vi "FTMS.vi"() -> ()   [LabVIEW 2012]
uses:
  Hardware Control/OSC/SubVIs/controls/sampling_rate.ctl
  Hardware Control/OSC/SubVIs/controls/scale.ctl
  global.vi
  <vilib>/Platform/browser.llb/Open URL in Default Browser (string).vi
panel:
  out "Meas Cycle \nDuration (s)":dbl=2.0 format="%.2g"
  out "Experiment \ncomplete in":string="00:00:00"
  out "Duration \nper Step":string="00:00:00"
  out "Time left for\ncurrent Step":string
  in  "about":bool
  in  "readme":bool
  out "Current Average":i32=2
  out "TRIG burst enable":bool=TRUE caption="Burst"
  out "TRIG inhibit off":dbl=0.000745 min=0.0 max=999.999999999995 format="%.1p"
  out "Writing File":bool
  out "OSC Reading":bool
  out "Waiting":bool
  out "Current Step":i32=4
  out "Current Center \nFrequency (Hz)":dbl=9000000000.0 format="%0.2p"
  in  "meas cluster":T1
  in  "Pause":bool
  in  "Stop":bool
  out "dt":dbl=2e-10 format="%#_6p"
  out "reset meas cycle timer":bool
  out "first start":bool
  in  "Tab Control":T2(tab)
  in  "Single Trigger":bool
  in  "EXP File Path":path=path "U:/Measurement Data" caption="Enter or select file path"
  in  "Safe Single Step Spectra":bool
  in  "Safe Single Step Time Signals":bool
  in  "Safe Combined Spectra":bool=TRUE
  in  "EXP Meas Period (s)":dbl=1.0 caption="Meas Period (s)" min=1.0 format="%.2g"
  in  "EXP Meas Cycles":i32=2 caption="Number of Averages" min=1 step=1
  out "Step Duration":string
  in  "Purge Freq.":dbl=2.0 caption="Purge Freq. (Hz)"
  in  "PURGE nozzle":bool
  out "TRIG BG cycle":dbl=0.001 caption="BG. cycle" min=0.0 max=999.999999999995 format="%.2p"
  out "TRIG mol delay":dbl=0.0006 caption="Mol. delay (s)" min=0.0 max=999.999999999995 format="%.2p"
  out "TRIG start time":dbl[](array[numeric])=[0.0, 1.1e-06, 6.6e-06, 6.4e-06] caption="Delay \nStarts (s)" format="%.3p"
  out "TRIG delay duration":dbl=4.7e-05 caption="Delay Cycle (s)" format="%.2p"
  out "TRIG duration":dbl[](array[numeric])=[5.65e-06, 5e-06, 4e-05, 5e-06] caption="Delay \nDurations (s)" min=0.0 format="%.3p"
  out "TRIG burst period":dbl=5e-05 caption="Burst Period (s)" format="%.2p"
  out "TRIG burst count":i32=3 caption="Bursts"
  in  "Refresh meas time":bool
  out "meas cycle time (ms)":u32
  out "OSC resolution":ext=25000.0 caption="Spectral Resolution (Hz)" format="%#_6p"
  out "OSC sample points":i32=200000 caption="Points / Frame"
  out "Horizontal Scale":T3=4e-06 items=["400ns/div"=4e-07, "1µs/div"=1e-06, "2µs/div"=2e-06, "4µs/div"=4e-06, "10µs/div"=1e-05, "20µs/div"=2e-05]
  out "meas duration (s)":dbl=3.9999999999999996e-05 format="%.1p"
  out "Sample Rate (Hz)":T4=5000000000.0 items=["20 GHz (50ps/sample)", "10 GHz (100ps/sample)", "5.0 GHz (200ps/sample)", "2.5 GHz (400ps/sample)", "1.25 GHz (0.8ns/sample)", "0.5 GHz (2ns/sample)"]
  in  "start experiment":bool
  in  "config TRIG":bool
  in  "config OSC":bool
  in  "PSG start freq":dbl=6000000000.0 caption="Start Freq. (Hz)" min=0.00025 max=67.0 step=1e-06 format="%#.12p"
  in  "PSG Amplitude1":dbl=10.0 caption="PSG1 Ampl (dBm)" min=-135.0 max=30.0 step=0.5 format="%#_8p"
  in  "PSG Amplitude 2":dbl=10.0 caption="PSG2 Ampl (dBm)" min=-135.0 max=30.0 step=0.5 format="%#_8p"
  in  "PSG freq offset":dbl=1500000000.0 caption="Freq. Offset (Hz)" min=0.00025 max=67.0 step=1e-06 format="%#.12p"
  in  "PSG steps":u32=4 caption="PSG Steps" min=1 step=1 format="%.0p"
  in  "PSG step size":dbl=1000000000.0 caption="Step Size" min=0.00025 max=67.0 step=1e-06 format="%#.12p"
  in  "write configs":bool
  in  "load config":bool
  in  "save config":bool
  in  "Save Config Info":bool
  in  "Date/Time in Path":bool
  in  "compound":string
  in  "Specific Path":bool
  out "date/time string":string
  out "Path Preview":path=path "U:/Measurement Data"
  out "Experiment Duration":string
  out "Cor Frame Time Signal":waveform(dbl)(graph)={"t0"=timestamp(0 s since 1904-01-01), "dt"=2e-10, "Y"=[]} caption="Corrected Frame Time Signal"
  out "BG Frame Time Signal":waveform(dbl)(graph)={"t0"=timestamp(0 s since 1904-01-01), "dt"=2e-10, "Y"=[]} caption="Background Frame Time Signal"
  out "Mol Frame Time Signal":waveform(dbl)(graph)={"t0"=timestamp(0 s since 1904-01-01), "dt"=2e-10, "Y"=[]} caption="Molecular Frame Time Signal"
  out "TD frame averages completed:":i32=2 caption="averages:"
  in  "frame FD single cycle":bool caption="no averaging"
  in  "reset TD frame ave":bool
  in  "TD Frame":i32=1 caption="Displayed Frame" min=1 step=1
  out "Mol Frame Spectra":T5(graph)={"Numeric Control"=10500000000.0, "df"=-24999.999999999996, "magnitude"=[]} caption="Molecular Frame Spectrum"
  out "BG Frame Spectra":T5(graph)={"Numeric Control"=10500000000.0, "df"=-24999.999999999996, "magnitude"=[]} caption="Background Frame Spectrum"
  out "Cor Frame Spectra":T5(graph)={"Numeric Control"=10500000000.0, "df"=-24999.999999999996, "magnitude"=[]} caption="Corrected Frame Spectrum"
  in  "Frame":i32=1 caption="Displayed Frame" min=1 step=1
  in  "reset frame average":bool
  in  "frame single cycle":bool caption="no averaging"
  out "frame averages completed:":i32=2 caption="averages:"
  out "TD Averaged Molecular":waveform(dbl)(graph)={"t0"=timestamp(0 s since 1904-01-01), "dt"=2e-10, "Y"=[]} caption="Averaged Time Signal - Molecular"
  out "TD Averaged Background":waveform(dbl)(graph)={"t0"=timestamp(0 s since 1904-01-01), "dt"=2e-10, "Y"=[]} caption="Averaged Time Signal - Background"
  out "TD Average Cor":waveform(dbl)(graph)={"t0"=timestamp(0 s since 1904-01-01), "dt"=2e-10, "Y"=[]} caption="Averaged Time Signal - Corrected"
  out "Average Cor":T5(graph)={"Numeric Control"=10500000000.0, "df"=-24999.999999999996, "magnitude"=[]} caption="Corrected - Average Spectrum"
  out "Averaged Background":T5(graph)={"Numeric Control"=10500000000.0, "df"=-24999.999999999996, "magnitude"=[]} caption="Background - Averaged Spectrum"
  out "Averaged Molecular":T5(graph)={"Numeric Control"=10500000000.0, "df"=-24999.999999999996, "magnitude"=[]} caption="Molecular Signal - Averaged Spectrum"
  out "combined spectra":T6(graph)
  in  "Show Complete":bool caption="Show All"
  in  "Quit":bool
  # "Chirped-Pulse Fourier Transform Microwave Spectroscopy"
  # "Experiment\nStatus"
  # "Timing Info"
  # "local variables"
  # "Software\nControl"
  # "General Settings"
  # "File Path"
  # "Select Data to Safe"
  # "OSC Configuration"
  # "TRIG Configuration"
  # "PSG Configuration"
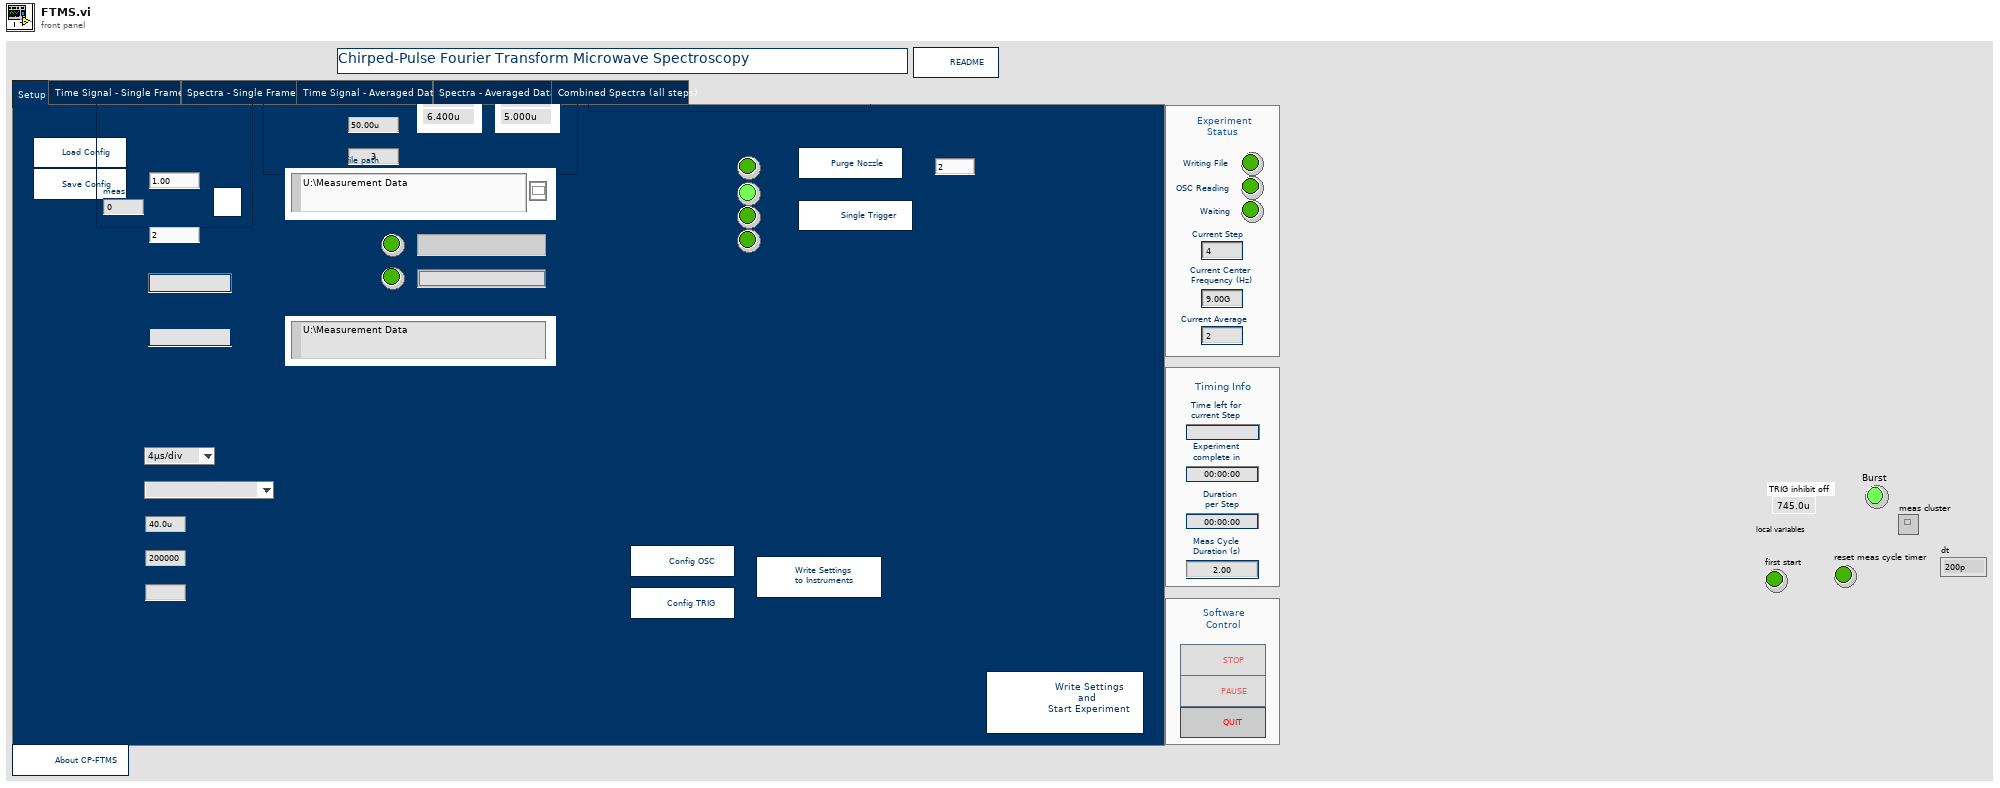
[diagram p1: front panel]
types:
  T1 = cluster{"spectra cluster":cluster{"BG spectrum":cluster{"Numeric Control":dbl, "df":dbl, "magnitude":dbl[]}, "Mol spectrum":cluster{"Numeric Control":dbl, "df":dbl, "magnitude":dbl[]}, "cor spectrum":cluster{"Numeric Control":dbl, "df":dbl, "magnitude":dbl[]}}, "time cluster":cluster{"cor waveform":waveform(dbl), "Mol waveform":waveform(dbl), "BG waveform":waveform(dbl)}}
  T2 = enum32{"Setup", "Time Signal - Single Frames", "Spectra - Single Frames", "Time Signal - Averaged Data", "Spectra - Averaged Data", "Combined Spectra (all steps)"}
  T3 = typedef "scale.ctl" = dbl
  T4 = typedef "sampling_rate.ctl" = ext
  T5 = cluster{"Numeric Control":dbl, "df":dbl, "magnitude":dbl[]}
  T6 = cluster{"Numeric Control":dbl, "df":dbl, "magnitude":dbl[]}[]
  T7 = enum8{"Enabled", "Disabled", "Disabled and Grayed Out"}
  T8 = enum16{"open", "replace", "create", "open or create", "replace or create", "replace or create with confirmation"}
  T9 = cluster{"cor waveform":waveform(dbl), "Mol waveform":waveform(dbl), "BG waveform":waveform(dbl)}
  T10 = cluster{"BG spectrum":cluster{"Numeric Control":dbl, "df":dbl, "magnitude":dbl[]}, "Mol spectrum":cluster{"Numeric Control":dbl, "df":dbl, "magnitude":dbl[]}, "cor spectrum":cluster{"Numeric Control":dbl, "df":dbl, "magnitude":dbl[]}}
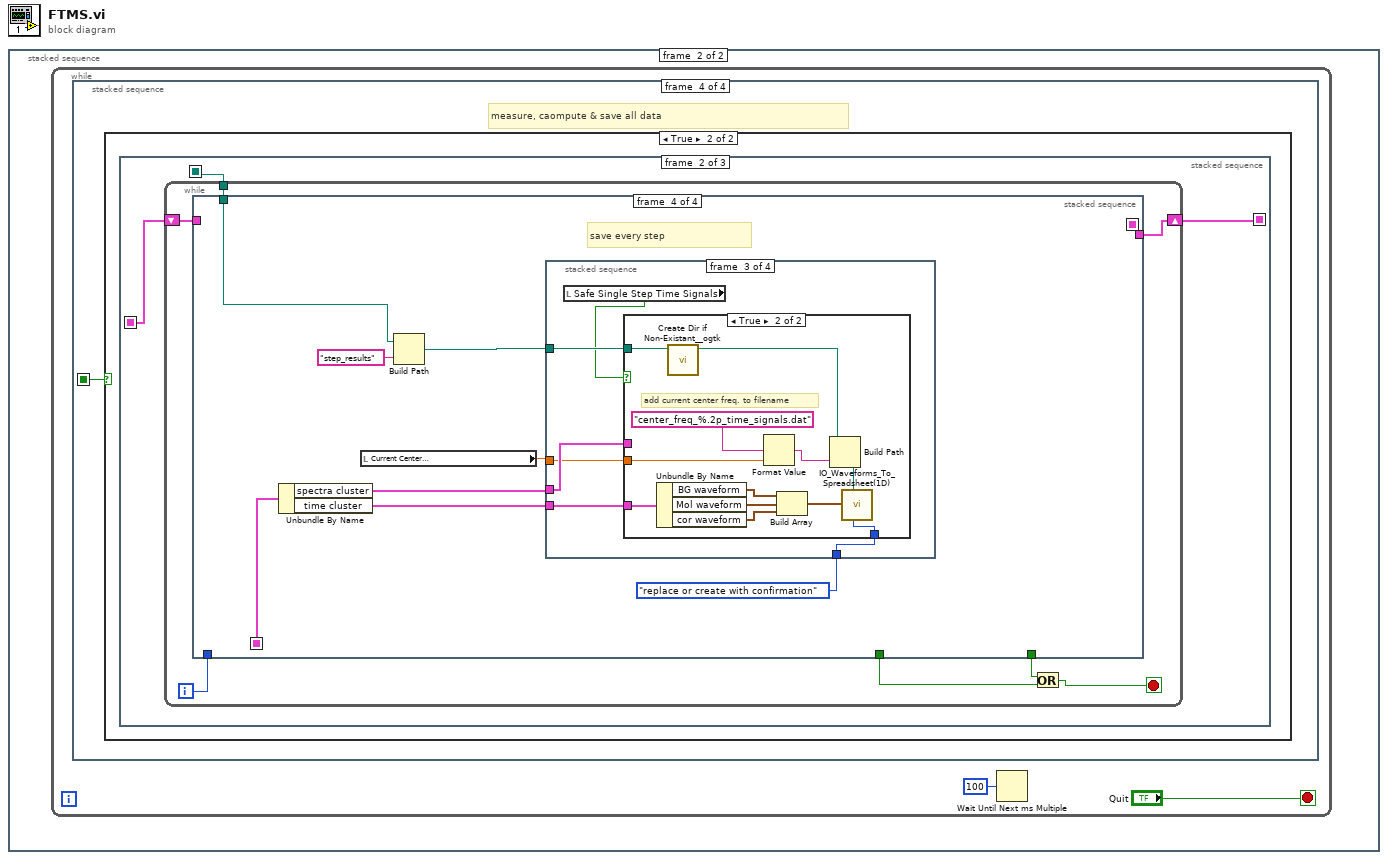
[diagram p0: block diagram]
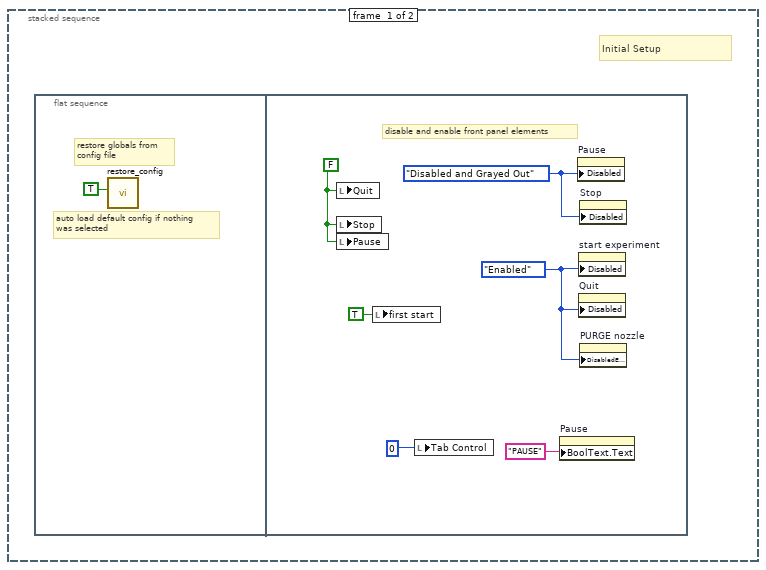
[diagram p2: hidden frame]
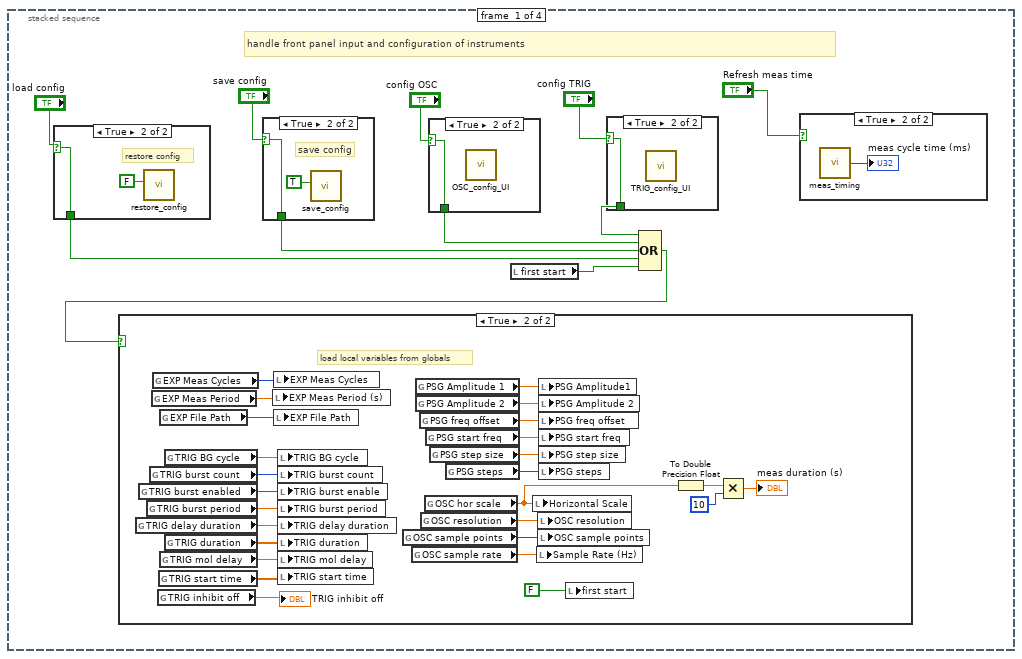
[diagram p3: hidden frame]
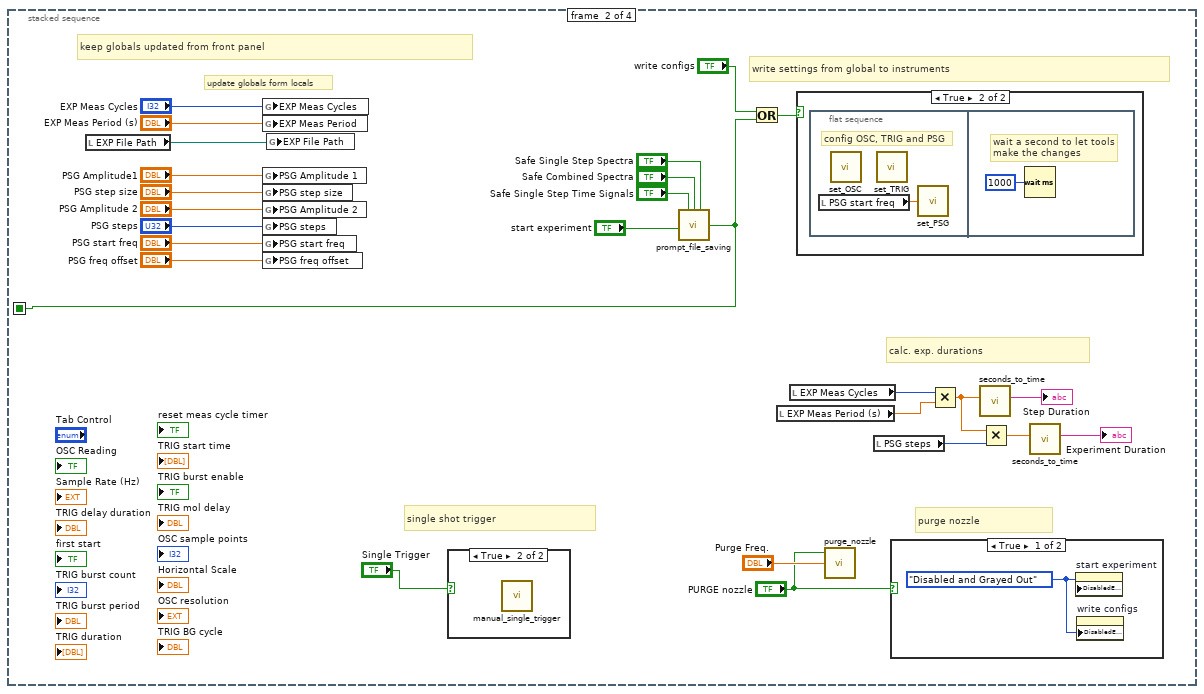
[diagram p10: hidden frame]
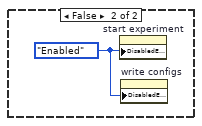
[diagram p12: hidden frame]
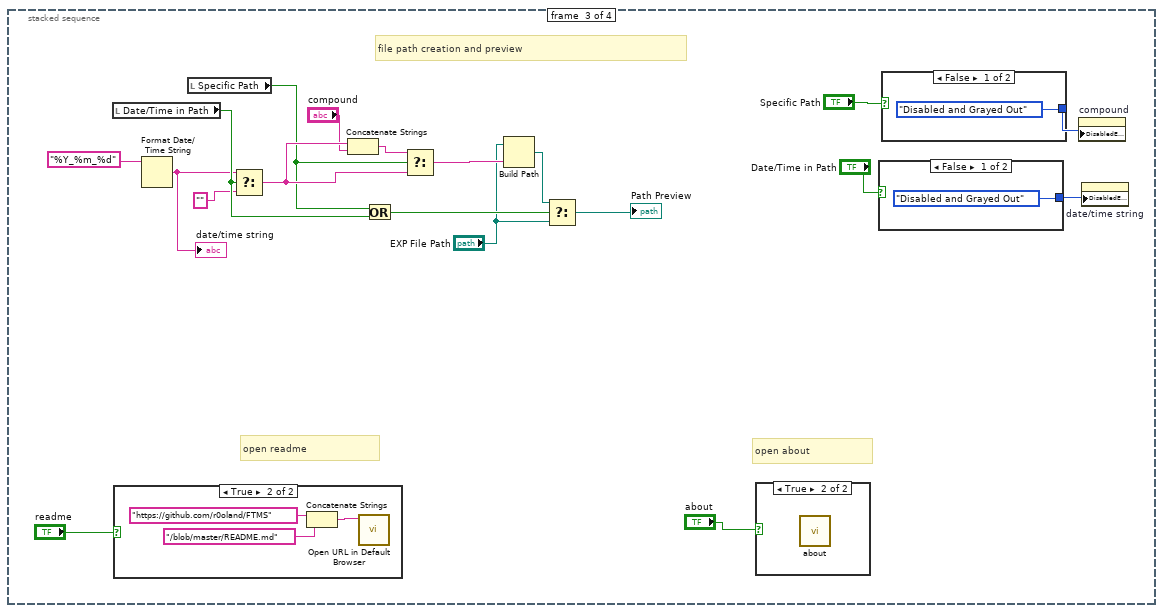
[diagram p14: hidden frame]
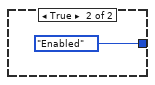
[diagram p17: hidden frame]
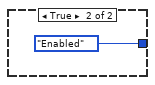
[diagram p18: hidden frame]
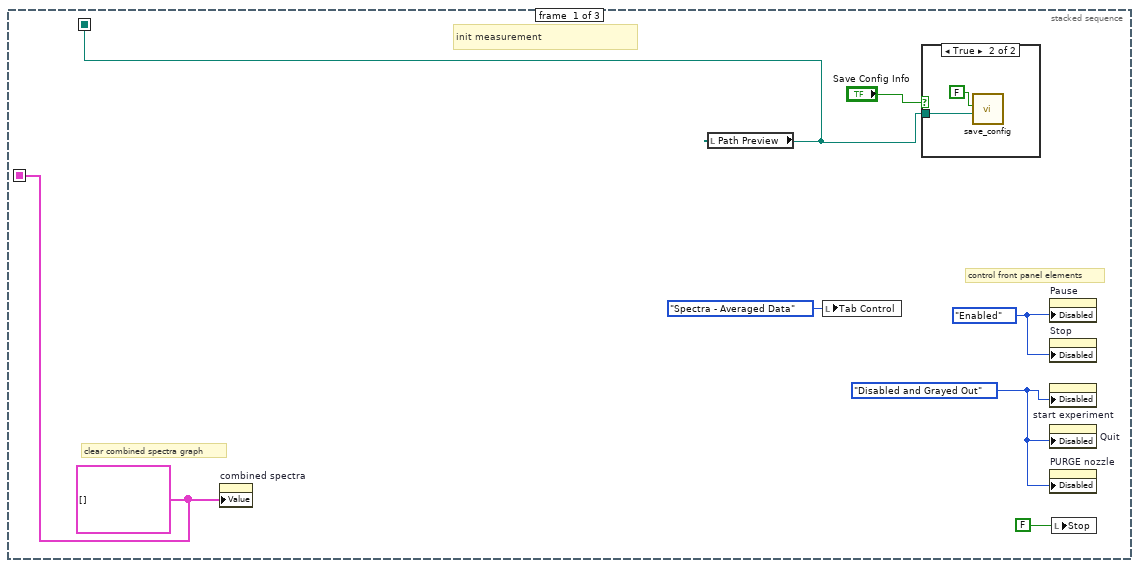
[diagram p20: hidden frame]
diagram:
  n1 = stacked-sequence {
    frame #0 {
      # "Initial Setup"
      n2 = flat-sequence {
        frame #0 {
          # "auto load default config if nothing\nwas selected"
          # "restore globals from\nconfig file"
          n3 = call "restore_config.vi"("Auto Load Default?"=TRUE) -> ()  [unwired: 4 in]
        }
        frame #1 {
          w6 = T7."Disabled and Grayed Out" ("Disabled")
          w2 = T7."Enabled" ("Disabled")
          w7 = FALSE ("Quit")
          # "disable and enable front panel elements"
          n4 = local write "Quit"(w7) -> ()
          n5 = local write "Stop"(w7) -> ()
          n6 = local write "Pause"(w7) -> ()
          n7 = local write "first start"(TRUE ("first start")) -> ()
          n8 = local write "Tab Control"(0) -> ()
          n9 = property on="Pause" class="Bool (strict)"("BoolText.Text"="PAUSE" ("Boolean Text.Text")) -> ()  [unwired: 2 in, 2 out]
          n10 = property on="Pause" class="Bool (strict)"("Disabled"=w6) -> ()  [unwired: 2 in, 2 out]
          n11 = property on="start experiment" class="Bool"("Disabled"=w2) -> ()  [unwired: 2 in, 2 out]
          n12 = property on="Quit" class="Bool (strict)"("Disabled"=w2) -> ()  [unwired: 2 in, 2 out]
          n13 = property on="Stop" class="Bool (strict)"("Disabled"=w6) -> ()  [unwired: 2 in, 2 out]
          n14 = property on="PURGE nozzle" class="Bool (strict)"("DisabledEnum"=w2) -> ()  [unwired: 2 in, 2 out]
        }
      }
    }
    frame #1 {
      n15 = while {
        stop <- "Quit" stop-if-true
        n16 = stacked-sequence {
          seq-local: [_ w63 _ _] -> [_ _ _ w114]
          frame #0 {
            # "handle front panel input and configuration of instruments"
            n17 = case shown="True" "load config" {
              selector: "load config" -> [w55 w57]
              tunnel: [w55 w57] -> w12
              frame False {
              }
              frame True {
                # "restore config"
                n18 = call "restore_config.vi"("Auto Load Default?"=FALSE) -> ()  [unwired: 4 in]
              }
            }
            n19 = case shown="True" "save config" {
              selector: "save config" -> [w52 w54]
              tunnel: [w52 w54] -> w14
              frame False {
              }
              frame True {
                # "save config"
                n20 = call "save_config.vi"("file dialog?"=TRUE) -> ()  [unwired: 4 in]
              }
            }
            n21 = case shown="True" "config OSC" {
              selector: "config OSC" -> [w50 w51]
              tunnel: [w50 w51] -> w16
              frame False {
              }
              frame True {
                n22 = call "OSC_config_UI.vi"() -> ()  [unwired: 12 in]
              }
            }
            n23 = local read "first start"() -> (w19:bool)
            n24 = case shown="True" "config TRIG" {
              selector: "config TRIG" -> [w48 w49]
              tunnel: [w48 w49] -> w17
              frame False {
              }
              frame True {
                n25 = call "TRIG_config_UI.vi"() -> ()  [unwired: 12 in]
              }
            }
            n26 = Compound Arithmetic op=OR(w17, w16, w14, w12, w19) -> (w11:bool)
            n27 = case shown="True" w11 {
              frame False {
              }
              frame True {
                # "load local variables from globals"
                n28 = global read "global.vi" "TRIG delay duration"() -> (w33:dbl)
                n29 = global read "global.vi" "TRIG burst enabled"() -> (w35:bool)
                n30 = global read "global.vi" "TRIG burst period"() -> (w34:dbl)
                n31 = global read "global.vi" "TRIG burst count"() -> (w36:i32)
                n32 = global read "global.vi" "EXP Meas Period"() -> (w28:dbl)
                n33 = global read "global.vi" "EXP Meas Cycles"() -> (w47:i32)
                n34 = global read "global.vi" "TRIG inhibit off"() -> (→"TRIG inhibit off":dbl)
                n35 = global read "global.vi" "TRIG start time"() -> (w30:dbl[])
                n36 = global read "global.vi" "EXP File Path"() -> (w22:path)
                n37 = global read "global.vi" "TRIG mol delay"() -> (w31:dbl)
                n38 = global read "global.vi" "TRIG BG cycle"() -> (w37:dbl)
                n39 = global read "global.vi" "TRIG duration"() -> (w32:dbl[])
                n40 = local write "EXP Meas Period (s)"(w28) -> ()
                n41 = local write "EXP Meas Cycles"(w47) -> ()
                n42 = local write "EXP File Path"(w22) -> ()
                n43 = local write "TRIG BG cycle"(w37) -> ()
                n44 = local write "TRIG burst count"(w36) -> ()
                n45 = local write "TRIG burst enable"(w35) -> ()
                n46 = local write "TRIG burst period"(w34) -> ()
                n47 = local write "TRIG delay duration"(w33) -> ()
                n48 = local write "TRIG duration"(w32) -> ()
                n49 = local write "TRIG mol delay"(w31) -> ()
                n50 = local write "TRIG start time"(w30) -> ()
                n51 = global read "global.vi" "OSC sample points"() -> (w45:i32)
                n52 = global read "global.vi" "OSC sample rate"() -> (w44:T4)
                n53 = global read "global.vi" "PSG Amplitude 1"() -> (w39:dbl)
                n54 = global read "global.vi" "PSG Amplitude 2"() -> (w40:dbl)
                n55 = global read "global.vi" "PSG freq offset"() -> (w41:dbl)
                n56 = global read "global.vi" "OSC resolution"() -> (w46:ext)
                n57 = global read "global.vi" "OSC hor scale"() -> (w24:T3)
                n58 = global read "global.vi" "PSG start freq"() -> (w42:dbl)
                n59 = global read "global.vi" "PSG step size"() -> (w43:dbl)
                n60 = global read "global.vi" "PSG steps"() -> (w38:i32)
                n61 = local write "Horizontal Scale"(w24) -> ()
                n62 = local write "Sample Rate (Hz)"(w44) -> ()
                n63 = local write "OSC resolution"(w46) -> ()
                n64 = local write "OSC sample points"(w45) -> ()
                n65 = local write "PSG Amplitude1"(w39) -> ()
                n66 = local write "PSG Amplitude 2"(w40) -> ()
                n67 = local write "PSG freq offset"(w41) -> ()
                n68 = local write "PSG start freq"(w42) -> ()
                n69 = local write "PSG step size"(w43) -> ()
                n70 = local write "PSG steps"(w38) -> ()
                n71 = local write "first start"(FALSE ("first start")) -> ()
                n72 = To Double Precision Float(number=w24) -> (double precision float=w26:T3)
                n73 = Multiply(x=w26, y=10) -> (x*y=→"meas duration (s)":T3)
              }
            }
            n74 = case shown="True" "Refresh meas time" {
              frame False {
              }
              frame True {
                n75 = call "meas_timing.vi"() -> ("meas cycle time"=→"meas cycle time (ms)":u32)  [unwired: 5 in]
              }
            }
          }
          frame #1 {
            # "single shot trigger"
            # "calc. exp. durations"
            # "purge nozzle"
            # "write settings from global to instruments"
            # "keep globals updated from front panel"
            # "update globals form locals"
            n76 = local read "EXP File Path"() -> (w64:path)
            n77 = global write "global.vi" "EXP Meas Cycles"("EXP Meas Cycles") -> ()
            n78 = global write "global.vi" "EXP Meas Period"("EXP Meas Period (s)") -> ()
            n79 = global write "global.vi" "PSG Amplitude 1"("PSG Amplitude1") -> ()
            n80 = global write "global.vi" "PSG step size"("PSG step size") -> ()
            n81 = global write "global.vi" "PSG Amplitude 2"("PSG Amplitude 2") -> ()
            n82 = global write "global.vi" "PSG steps"("PSG steps") -> ()
            n83 = global write "global.vi" "PSG start freq"("PSG start freq") -> ()
            n84 = global write "global.vi" "PSG freq offset"("PSG freq offset") -> ()
            n85 = global write "global.vi" "EXP File Path"(w64) -> ()
            n86 = case shown="True" "Single Trigger" {
              frame False {
              }
              frame True {
                n87 = call "manual_single_trigger.vi"() -> ()  [unwired: 12 in]
              }
            }
            n88 = call "prompt_file_saving.vi"("safe time steps"="Safe Single Step Time Signals", "safe combined spectra"="Safe Combined Spectra", "safe spectra steps"="Safe Single Step Spectra", "start exp"="start experiment") -> ("Start Experiment"=w63:bool)  [unwired: 11 in]
            n89 = Or(x="write configs", y=w63) -> (x .or. y?=w75:bool)
            n90 = local read "EXP Meas Period (s)"() -> (w70:dbl)
            n91 = local read "EXP Meas Cycles"() -> (w71:i32)
            n92 = case shown="True" w75 {
              frame False {
              }
              frame True {
                n93 = flat-sequence {
                  frame #0 {
                    # "config OSC, TRIG and PSG"
                    n94 = local read "PSG start freq"() -> (w86:dbl)
                    n95 = call "set_OSC.vi"() -> ()  [unwired: 12 in]
                    n96 = call "set_TRIG.vi"() -> ()  [unwired: 12 in]
                    n97 = call "set_PSG.vi"("PSG1 frequency"=w86) -> ()  [unwired: 5 in]
                  }
                  frame #1 {
                    # "wait a second to let tools \nmake the changes"
                    n98 = Wait (ms)(milliseconds to wait=u32 1000) -> ()  [unwired: 1 out]
                  }
                }
              }
            }
            n99 = call "purge_nozzle.vi"("purge frequency"="Purge Freq.", "Purge"="PURGE nozzle") -> ()  [unwired: 4 in]
            n100 = local read "PSG steps"() -> (w67:u32)
            n101 = case shown="True" "PURGE nozzle" {
              frame True {
                w84 = T7."Disabled and Grayed Out" ("Disabled")
                n102 = property on="start experiment" class="Bool"("DisabledEnum"=w84) -> ()  [unwired: 2 in, 2 out]
                n103 = property on="write configs" class="Bool"("DisabledEnum"=w84) -> ()  [unwired: 2 in, 2 out]
              }
              frame False {
                w85 = T7."Enabled" ("Disabled")
                n104 = property on="start experiment" class="Bool"("DisabledEnum"=w85) -> ()  [unwired: 2 in, 2 out]
                n105 = property on="write configs" class="Bool"("DisabledEnum"=w85) -> ()  [unwired: 2 in, 2 out]
              }
            }
            n106 = Multiply(x=w71, y=w70) -> (x*y=w68:dbl)
            n107 = call "seconds_to_time.vi"("# Seconds (0)"=w68) -> ("Elapsed Time (00:00:00)"=→"Step Duration":string)  [unwired: 10 in]
            n108 = Multiply(x=w68, y=w67) -> (x*y=w65:dbl)
            n109 = call "seconds_to_time.vi"("# Seconds (0)"=w65) -> ("Elapsed Time (00:00:00)"=→"Experiment Duration":string)  [unwired: 10 in]
          }
          frame #2 {
            # "open about"
            # "open readme"
            # "file path creation and preview"
            n110 = local read "Date/Time in Path"() -> (w97:bool)
            n111 = case shown="True" "readme" {
              frame False {
              }
              frame True {
                n112 = Concatenate Strings("https://github.com/r0oland/FTMS" ("string"), "/blob/master/README.md" ("string")) -> (w109:string)
                n113 = call-poly <vilib>:"Open URL in Default Browser.vi"("URL"=w109) -> ()  [unwired: 5 in, 2 out]
              }
            }
            n114 = Format Date/Time String(time format string (%c)="%Y_%m_%d") -> (date/time string=w90:string)  [unwired: 2 in]
            "date/time string" <- w90
            n115 = local read "Specific Path"() -> (w98:bool)
            n116 = Select(t=w90, s=w97, f="") -> (s? t:f=w101:string)
            n117 = Concatenate Strings(w101, "compound") -> (w100:string)
            n118 = Or(x=w98, y=w97) -> (x .or. y?=w95:bool)
            n119 = Select(t=w100, s=w98, f=w101) -> (s? t:f=w94:string)
            n120 = Build Path(base path="EXP File Path", name or relative path=w94) -> (appended path=w92:path)
            n121 = Select(t=w92, s=w95, f="EXP File Path") -> (s? t:f=→"Path Preview":path)
            n122 = case shown="True" "about" {
              frame False {
              }
              frame True {
                n123 = call "about.vi"() -> ()  [unwired: 12 in]
              }
            }
            n124 = case shown="False" "Date/Time in Path" {
              tunnel: [T7."Disabled and Grayed Out" ("Disabled") T7."Enabled" ("Disabled")] -> w104
              frame False {
              }
              frame True {
              }
            }
            n125 = case shown="False" "Specific Path" {
              tunnel: [T7."Disabled and Grayed Out" ("Disabled") T7."Enabled" ("Disabled")] -> w105
              frame False {
              }
              frame True {
              }
            }
            n126 = property on="compound" class="Str"("DisabledEnum"=w105) -> ()  [unwired: 2 in, 2 out]
            n127 = property on="date/time string" class="Str"("DisabledEnum"=w104) -> ()  [unwired: 2 in, 2 out]
          }
          frame #3 {
            # "measure, caompute & save all data"
            n128 = case shown="True" w114 {
              frame False {
              }
              frame True {
                n129 = stacked-sequence {
                  seq-local: [w116 _ _] -> [_ w126 w326]
                  seq-local: [_ w125 _] -> [_ _ w328]
                  seq-local: [w118 _ _] -> [_ w124 _]
                  frame #0 {
                    w118 = T6 [] ("combined spectra")
                    w121 = T7."Enabled" ("Disabled")
                    w120 = T7."Disabled and Grayed Out" ("Disabled")
                    # "clear combined spectra graph"
                    # "init measurement"
                    # "control front panel elements"
                    n130 = property on="combined spectra" class="WFGraph (strict)"("Value"=w118) -> ()  [unwired: 2 in, 2 out]
                    n131 = local read "Path Preview"() -> (w116:path)
                    n132 = local write "Tab Control"(T2."Spectra - Averaged Data" ("Tab Control")) -> ()
                    n133 = case shown="True" "Save Config Info" {
                      tunnel: w116 -> [_ w122]
                      frame False {
                      }
                      frame True {
                        n134 = call "save_config.vi"("selected path"=w122, "file dialog?"=FALSE) -> ()  [unwired: 3 in]
                      }
                    }
                    n135 = property on="Pause" class="Bool (strict)"("Disabled"=w121) -> ()  [unwired: 2 in, 2 out]
                    n136 = property on="Stop" class="Bool (strict)"("Disabled"=w121) -> ()  [unwired: 2 in, 2 out]
                    n137 = property on="start experiment" class="Bool"("Disabled"=w120) -> ()  [unwired: 2 in, 2 out]
                    n138 = property on="Quit" class="Bool (strict)"("Disabled"=w120) -> ()  [unwired: 2 in, 2 out]
                    n139 = property on="PURGE nozzle" class="Bool (strict)"("Disabled"=w120) -> ()  [unwired: 2 in, 2 out]
                    n140 = local write "Stop"(FALSE ("Stop")) -> ()
                  }
                  frame #1 {
                    n141 = while {
                      tunnel: w126 -> [w129]
                      shift-right: [w127] -> w125
                      shift-left: w124 -> [w128]
                      i -> [w133]
                      stop <- w131 stop-if-true
                      n142 = stacked-sequence {
                        seq-local: [_ w148 _ _] -> [_ _ _ w286]
                        seq-local: [_ w146 _ _] -> [_ _ w275 _]
                        tunnel: w133 -> [w138 _ _ _]
                        tunnel: [w137 _ _ _] -> w132
                        tunnel: [_ w150 _ _] -> w130
                        tunnel: w129 -> [_ _ _ w282]
                        tunnel: w128 -> [_ w145 _ _]
                        tunnel: [_ _ w275 _] -> w127
                        frame #0 {
                          # "stop after specific number of steps"
                          # "freq. settings for specific step"
                          n143 = global read "global.vi" "PSG step size"() -> (w141:dbl)
                          n144 = local read "PSG start freq"() -> (w140:dbl)
                          n145 = Increment(x=w138) -> (x+1=w135:i32)
                          "Current Step" <- w135
                          n146 = Multiply(x=w141, y=w138) -> (x*y=w139:dbl)
                          n147 = Add(x=w140, y=w139) -> (x+y=w134:dbl)
                          "Current Center \nFrequency (Hz)" <- w134
                          n148 = flat-sequence {
                            tunnel: w134 -> [w143]
                            frame #0 {
                              # "turn off RF"
                              n149 = call "output_on_PSG.vi"("Enable RF Output (F:Disable)"=FALSE) -> ()  [unwired: 5 in]
                            }
                            frame #1 {
                              n150 = call "set_PSG.vi"("PSG1 frequency"=w143) -> ()  [unwired: 5 in]
                            }
                            frame #2 {
                              # "turn on RF"
                              n151 = call "output_on_PSG.vi"("Enable RF Output (F:Disable)"=TRUE) -> ()  [unwired: 5 in]
                            }
                          }
                          n152 = global read "global.vi" "PSG steps"() -> (w136:i32)
                          n153 = Greater Or Equal?(x=w135, y=w136) -> (x >= y?=w137:bool)
                        }
                        frame #1 {
                          # "acquire & dispaly single spectra"
                          n154 = call "get_acq_number.vi"("reset acq. number?"=TRUE) -> ("# of meas cycles"=w151:i32)  [unwired: 7 in, 3 out]
                          n155 = while {
                            tunnel: w151 -> [w161]
                            shift-right: [w159] -> _
                            shift-left: 0.0 -> [w158]
                            tunnel: ["Stop"] -> w150
                            tunnel: [w155] -> w148
                            tunnel: [w154] -> w147
                            tunnel: w145 -> [w153]
                            i -> [w162]
                            stop <- w157 stop-if-true
                            n156 = stacked-sequence {
                              seq-local: [_ _ w187 _ _ _ _ _ _ _] -> [_ _ _ w200 w209 w228 w237 _ _ _]
                              seq-local: [w163 _ _ _ _ _ _ _ _ _] -> [_ _ _ _ _ _ _ w262 _ _]
                              tunnel: w162 -> [_ _ _ w205 w219 w233 w251 _ _ _]
                              tunnel: w161 -> [w167 _ _ _ _ _ _ _ _ w273]
                              tunnel: [_ _ _ _ _ _ _ _ _ w270] -> w160
                              tunnel: [_ w171 _ _ _ _ _ _ _ _] -> w159
                              tunnel: w158 -> [_ w170 _ _ _ _ _ _ _ _]
                              tunnel: [_ _ _ _ _ _ w239 _ _ _] -> w155
                              tunnel: [_ _ _ _ _ _ w238 _ _ _] -> w154
                              tunnel: w153 -> [_ _ _ _ _ _ _ _ w264 _]
                              frame #0 {
                                # "display current meas cylce"
                                n157 = Tick Count (ms)() -> (millisecond timer value=w163:u32)
                                n158 = call "get_acq_number.vi"("reset acq. number?"=FALSE) -> ("# of meas cycles"=w168:i32)  [unwired: 7 in, 3 out]
                                n159 = Subtract(x=w168, y=w167) -> (x-y=w165:i32)
                                n160 = Increment(x=w165) -> (x+1=→"Current Average":i32)
                              }
                              frame #1 {
                                n161 = while {
                                tunnel: [w179] -> w171
                                tunnel: w170 -> [w185]
                                tunnel: ["Pause"] -> w169
                                stop <- w181 stop-if-true
                                n162 = global read "global.vi" "EXP Meas Period"() -> (w183:dbl)
                                n163 = Get Date/Time In Seconds() -> (seconds since 1Jan1904=w186:timestamp)
                                n164 = To Double Precision Float(number=w186) -> (double precision float=w179:dbl)
                                n165 = Subtract(x=w179, y=w185) -> (x-y=w184:dbl)
                                n166 = Greater?(x=w184, y=w183) -> (0:w178:bool)
                                n167 = Not(x="Pause") -> (.not. x?=w177:bool)
                                n168 = And(x=w178, y=w177) -> (x .and. y?=w181:bool)
                                n169 = Not(x=w181) -> (.not. x?=→"Waiting":bool)
                                n170 = Wait (ms)(milliseconds to wait=u32 10) -> ()  [unwired: 1 out]
                                }
                                n171 = case shown="True" w169 {
                                frame False {
                                n172 = property on="Stop" class="Bool (strict)"("DisabledEnum"=T7."Enabled" ("Disabled")) -> ()  [unwired: 2 in, 2 out]
                                n173 = property on="Pause" class="Bool (strict)"("BoolText.Text"="Pause" ("Caption.Text")) -> ()  [unwired: 2 in, 2 out]
                                }
                                frame True {
                                n174 = property on="Pause" class="Bool (strict)"("BoolText.Text"="Resume" ("Caption.Text")) -> ()  [unwired: 2 in, 2 out]
                                n175 = property on="Stop" class="Bool (strict)"("DisabledEnum"=T7."Disabled and Grayed Out" ("Disabled")) -> ()  [unwired: 2 in, 2 out]
                                }
                                }
                              }
                              frame #2 {
                                n176 = flat-sequence {
                                tunnel: [w191] -> w187
                                frame #0 {
                                n177 = local write "OSC Reading"(TRUE) -> ()
                                }
                                frame #1 {
                                w190 = u16 0 items=["Channel 1", "Channel 2", "Channel 3", "Channel 4", "Math 1", "Math 2", "Math 3", "Math 4", "Reference 1", "Reference 2", "Reference 3", "Reference 4"] ("Channel (0: Channel 1)")
                                # "trigger OSC and read waveform"
                                n178 = call "read_OSC.vi"("Channel (0: Channel 1)"=w190) -> ("3D waveform array"=w191:dbl[][][], "dt"=→"dt":dbl)  [unwired: 4 in, 5 out]
                                }
                                frame #2 {
                                n179 = local write "OSC Reading"(FALSE) -> ()
                                }
                                }
                              }
                              frame #3 {
                                # "reset on first frame"
                                # "display frame time info"
                                n180 = local read "Current Center \nFrequency (Hz)"() -> (w207:dbl)
                                n181 = local read "PSG freq offset"() -> (w201:dbl)
                                n182 = Equal?(x=0, y=w205) -> (x = y?=w203:bool)
                                n183 = local read "dt"() -> (w208:dbl)
                                n184 = Compound Arithmetic op=OR("frame FD single cycle", w203, "reset TD frame ave") -> (w202:bool)
                                n185 = call "FFT_averaging.vi"("dt"=w208, "freq. offset"=w201, "frame"="TD Frame", "current frequency"=w207, "3d waveform array"=w200, "reset frame average"=w202, "all frames?"=FALSE) -> ("BG waveform"=→"BG Frame Time Signal":waveform(dbl), "Mol waveform"=→"Mol Frame Time Signal":waveform(dbl), "averages compl"=→"TD frame averages completed:":i32, "cor waveform"=→"Cor Frame Time Signal":waveform(dbl))  [unwired: 6 in, 3 out]
                              }
                              frame #4 {
                                # "reset on first frame"
                                # "display frame spectra"
                                n186 = local read "Current Center \nFrequency (Hz)"() -> (w223:dbl)
                                n187 = local read "PSG freq offset"() -> (w210:dbl)
                                n188 = Equal?(x=0, y=w219) -> (x = y?=w216:bool)
                                n189 = local read "dt"() -> (w224:dbl)
                                n190 = Compound Arithmetic op=OR("reset frame average", w216, "frame single cycle") -> (w214:bool)
                                n191 = call "FFT_averaging.vi"("dt"=w224, "freq. offset"=w210, "frame"="Frame", "current frequency"=w223, "3d waveform array"=w209, "reset frame average"=w214, "all frames?"=FALSE) -> ("averages compl"=→"frame averages completed:":i32, "BG spectrum"=→"BG Frame Spectra":T5, "Mol spectrum"=→"Mol Frame Spectra":T5, "cor spectrum"=→"Cor Frame Spectra":T5)  [unwired: 6 in, 3 out]
                              }
                              frame #5 {
                                # "reset only on first meas cycle"
                                # "display time signals averaged over all frames and over all meas cycles"
                                n192 = local read "Current Center \nFrequency (Hz)"() -> (w231:dbl)
                                n193 = Equal?(x=0, y=w233) -> (x = y?=w230:bool)
                                n194 = local read "PSG freq offset"() -> (w229:dbl)
                                n195 = local read "dt"() -> (w232:dbl)
                                n196 = call "FFT_averaging.vi"("dt"=w232, "freq. offset"=w229, "current frequency"=w231, "3d waveform array"=w228, "reset frame average"=w230, "all frames?"=TRUE) -> ("BG waveform"=→"TD Averaged Background":waveform(dbl), "Mol waveform"=→"TD Averaged Molecular":waveform(dbl), "cor waveform"=→"TD Average Cor":waveform(dbl))  [unwired: 7 in, 4 out]
                              }
                              frame #6 {
                                # "combine data for saving"
                                # "reset only on first meas cycle"
                                # "display spectra averaged over all frames and over all meas cycles"
                                n197 = local read "Current Center \nFrequency (Hz)"() -> (w249:dbl)
                                n198 = Equal?(x=0, y=w251) -> (x = y?=w248:bool)
                                n199 = local read "PSG freq offset"() -> (w240:dbl)
                                n200 = local read "dt"() -> (w250:dbl)
                                n201 = call "FFT_averaging.vi"("dt"=w250, "freq. offset"=w240, "current frequency"=w249, "3d waveform array"=w237, "reset frame average"=w248, "all frames?"=TRUE) -> ("BG waveform"=w243:waveform(dbl), "Mol waveform"=w244:waveform(dbl), "cor waveform"=w245:waveform(dbl), "BG spectrum"=w247:T5, "Mol spectrum"=w246:T5, "cor spectrum"=w238:T5)  [unwired: 7 in, 1 out]
                                "Average Cor" <- w238
                                "Averaged Background" <- w247
                                "Averaged Molecular" <- w246
                                n202 = Bundle("cor waveform"=w245, "Mol waveform"=w244, "BG waveform"=w243) -> (w236:T9)  [unwired: 1 in]
                                n203 = Bundle ("bundle time domain data")("BG spectrum"=w247, "Mol spectrum"=w246, "cor spectrum"=w238) -> (w241:T10)  [unwired: 1 in]
                                n204 = Bundle By Name(cluster="meas cluster", "spectra cluster"=w241, "time cluster"=w236) -> (w239:T1)
                              }
                              frame #7 {
                                # "display time left"
                                n205 = Tick Count (ms)() -> (millisecond timer value=w261:u32)
                                n206 = Subtract(x=w261, y=w262) -> (x-y=w256:u32)
                                n207 = local read "Current Average"() -> (w255:i32)
                                n208 = local read "Current Step"() -> (w260:i32)
                                n209 = call "average_meas_duration.vi"("current meas cycle"=w255, "current step"=w260, "time diff (ms)"=w256) -> ("time for this step"=→"Time left for\ncurrent Step":string, "step duration"=→"Duration \nper Step":string, "time left for exp"=→"Experiment \ncomplete in":string, "meas cycle \nduration (s)"=→"Meas Cycle \nDuration (s)":dbl)
                              }
                              frame #8 {
                                n210 = case shown="True" "Show Complete" {
                                tunnel: w264 -> [_ w266]
                                frame False {
                                }
                                frame True {
                                n211 = local read "PSG freq offset"() -> (w265:dbl)
                                n212 = call "find_max_min_freq_in_spectra_cluster.vi"("Array"=w266, "freq offset"=w265) -> ("min freq"=w267:dbl, "max freq"=w268:dbl)  [unwired: 2 in]
                                n213 = property on="combined spectra" class="WFGraph (strict)"("XScale.Maximum"=w268, "XScale.Minimum"=w267) -> ()  [unwired: 2 in, 2 out]
                                }
                                }
                              }
                              frame #9 {
                                # "stop after N measurments"
                                n214 = global read "global.vi" "EXP Meas Cycles"() -> (w271:i32)
                                n215 = call "get_acq_number.vi"("reset acq. number?"=FALSE) -> ("# of meas cycles"=w274:i32)  [unwired: 7 in, 3 out]
                                n216 = Subtract(x=w274, y=w273) -> (x-y=w269:i32)
                                n217 = Greater Or Equal?(x=w269, y=w271) -> (x >= y?=w270:bool)
                              }
                            }
                            n218 = Or(x=w160, y="Stop") -> (x .or. y?=w157:bool)
                          }
                          n219 = Build Array (concatenate)(w145, w147) -> (w146:T6)
                        }
                        frame #2 {
                          # "display combined spectra"
                          # "automatic scaling seems not to work, hence do it manually for the combined result."
                          # "display combined spectra"
                          n220 = local read "PSG freq offset"() -> (w278:dbl)
                          n221 = call "find_max_min_freq_in_spectra_cluster.vi"("Array"=w275, "freq offset"=w278) -> ("min freq"=w276:dbl, "max freq"=w277:dbl)  [unwired: 2 in]
                          n222 = property on="combined spectra" class="WFGraph (strict)"("XScale.Maximum"=w277, "XScale.Minimum"=w276) -> ()  [unwired: 2 in, 2 out]
                          "combined spectra" <- w275
                        }
                        frame #3 {
                          # "save every step"
                          n223 = Unbundle By Name(w286) -> ("spectra cluster"=w285:T10, "time cluster"=w284:T9)
                          n224 = local read "Current Center \nFrequency (Hz)"() -> (w281:dbl)
                          n225 = Build Path(base path=w282, name or relative path="step_results") -> (appended path=w280:path)
                          n226 = stacked-sequence {
                            tunnel: w285 -> [_ w290 w310 _]
                            tunnel: w284 -> [_ _ w309 _]
                            tunnel: w280 -> [_ w291 w308 _]
                            tunnel: w281 -> [_ w292 w307 _]
                            tunnel: T8."replace or create with confirmation" ("operation (0:open)") -> [_ w288 w305 _]
                            frame #0 {
                              "Writing File" <- TRUE
                            }
                            frame #1 {
                              n227 = local read "Safe Single Step Spectra"() -> (w289:bool)
                              n228 = case shown="True" w289 {
                                tunnel: w291 -> [_ w295]
                                tunnel: w292 -> [_ w303]
                                tunnel: w290 -> [_ w301]
                                tunnel: w288 -> [_ w293]
                                frame False {
                                }
                                frame True {
                                # "add current center freq. to filename"
                                n229 = Unbundle By Name(w301) -> ("BG spectrum"=w300:T5, "Mol spectrum"=w299:T5, "cor spectrum"=w298:T5)
                                n230 = call "Create Dir if Non-Existant__ogtk.vi"("Directory Path"=w295) -> ("dup Directory Path"=w294:path)  [unwired: 8 in, 2 out]
                                n231 = Build Array(w300, w299, w298) -> (w296:T6)
                                n232 = Format Value(format string="center_freq_%.2p_spectra.dat", value (0)=w303) -> (output string=w302:string)  [unwired: 1 in]
                                n233 = Build Path(base path=w294, name or relative path=w302) -> (appended path=w297:path)
                                n234 = call "IO_Export_Spectra_To_Spreadsheet.vi"("operation (0:open)"=w293, "Array 2"=w296, "file path (dialog if empty)"=w297) -> ()  [unwired: 9 in]
                                }
                              }
                            }
                            frame #2 {
                              n235 = local read "Safe Single Step Time Signals"() -> (w306:bool)
                              n236 = case shown="True" w306 {
                                tunnel: w310 -> [_ _]
                                tunnel: w309 -> [_ w322]
                                tunnel: w308 -> [_ w315]
                                tunnel: w307 -> [_ w317]
                                tunnel: w305 -> [_ w311]
                                frame False {
                                }
                                frame True {
                                # "add current center freq. to filename"
                                n237 = Unbundle By Name(w322) -> ("BG waveform"=w321:waveform(dbl), "Mol waveform"=w320:waveform(dbl), "cor waveform"=w319:waveform(dbl))
                                n238 = call "Create Dir if Non-Existant__ogtk.vi"("Directory Path"=w315) -> ("dup Directory Path"=w314:path)  [unwired: 8 in, 2 out]
                                n239 = Format Value(format string="center_freq_%.2p_time_signals.dat", value (0)=w317) -> (output string=w316:string)  [unwired: 1 in]
                                n240 = Build Array(w321, w320, w319) -> (w312:waveform(dbl)[])
                                n241 = Build Path(base path=w314, name or relative path=w316) -> (appended path=w313:path)
                                n242 = call "IO_Waveforms_To_Spreadsheet(1D).vi"("operation (0:open)"=w311, "waveforms"=w312, "file path (dialog if empty)"=w313) -> ()  [unwired: 8 in, 1 out]
                                }
                              }
                            }
                            frame #3 {
                              n243 = local write "Writing File"(FALSE) -> ()
                            }
                          }
                        }
                      }
                      n244 = Or(x=w132, y=w130) -> (x .or. y?=w131:bool)
                    }
                  }
                  frame #2 {
                    w327 = FALSE ("Stop")
                    w331 = T7."Disabled and Grayed Out" ("Disabled")
                    w330 = T7."Enabled" ("Disabled")
                    # "save combined spectra"
                    # "turn off RF"
                    n245 = local write "Stop"(w327) -> ()
                    n246 = local write "Pause"(w327) -> ()
                    n247 = local write "PURGE nozzle"(w327) -> ()
                    n248 = call "output_on_PSG.vi"("Enable RF Output (F:Disable)"=FALSE) -> ()  [unwired: 5 in]
                    n249 = property on="Pause" class="Bool (strict)"("Disabled"=w331) -> ()  [unwired: 2 in, 2 out]
                    n250 = property on="Stop" class="Bool (strict)"("Disabled"=w331) -> ()  [unwired: 2 in, 2 out]
                    n251 = property on="start experiment" class="Bool"("Disabled"=w330) -> ()  [unwired: 2 in, 2 out]
                    n252 = property on="Quit" class="Bool (strict)"("Disabled"=w330) -> ()  [unwired: 2 in, 2 out]
                    n253 = property on="PURGE nozzle" class="Bool (strict)"("Disabled"=w330) -> ()  [unwired: 2 in, 2 out]
                    n254 = local write "Tab Control"(T2."Combined Spectra (all steps)" ("Tab Control")) -> ()
                    n255 = local read "Safe Combined Spectra"() -> (w325:bool)
                    n256 = case shown="True" w325 {
                      selector: w325 -> [_ w337]
                      tunnel: w328 -> [_ w338]
                      tunnel: w326 -> [_ w335]
                      frame False {
                      }
                      frame True {
                        n257 = call "Create Dir if Non-Existant__ogtk.vi"("Directory Path"=w335) -> ("dup Directory Path"=w334:path)  [unwired: 8 in, 2 out]
                        n258 = Build Path(base path=w334, name or relative path="combined_results.dat") -> (appended path=w333:path)
                        n259 = stacked-sequence {
                          tunnel: w337 -> [w339 w341 _]
                          tunnel: w338 -> [_ w343 _]
                          tunnel: w333 -> [_ w342 _]
                          tunnel: T8."replace or create with confirmation" ("operation (0:open)") -> [_ w340 _]
                          frame #0 {
                            n260 = local write "Writing File"(w339) -> ()
                          }
                          frame #1 {
                            n261 = call "IO_Export_Spectra_To_Spreadsheet.vi"("operation (0:open)"=w340, "multiple time columns? (single:F)"=w341, "Array 2"=w343, "file path (dialog if empty)"=w342) -> ()  [unwired: 8 in]
                          }
                          frame #2 {
                            n262 = local write "Writing File"(FALSE) -> ()
                          }
                        }
                      }
                    }
                  }
                }
              }
            }
          }
        }
        n263 = Wait Until Next ms Multiple(millisecond multiple=u32 100) -> ()  [unwired: 1 out]
      }
    }
  }
